vi "Substitute the assigned name for Test UI.vi"(8 "error in":errorcluster, 10 "Project Name":string, 11 "Name to VI Map":map{string, refnum<vi>}(c390)) -> (0 "error out":errorcluster)   [LabVIEW 2023, in "Plugin Generator.lvlib"]
uses:
  Plugin Generator.lvlib
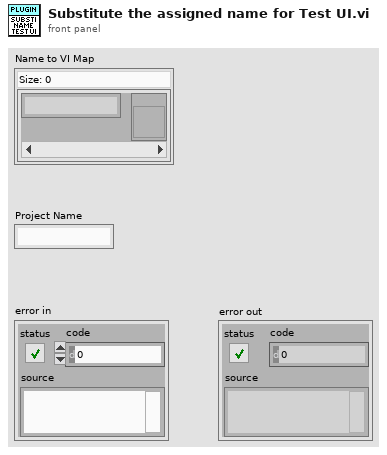
[diagram p1: front panel]
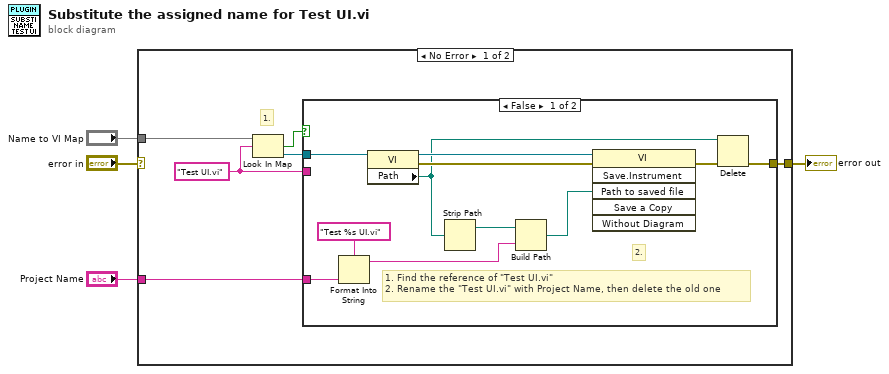
[diagram p0: block diagram]
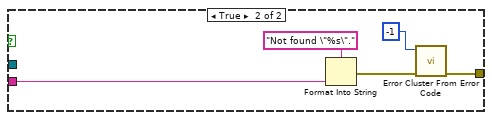
[diagram p2: hidden frame]
diagram:
  n1 = case shown="No Error" "error in" {
    selector: "error in" -> [_ w27]
    tunnel: "Project Name" -> [w10 _]
    tunnel: [w9 w27] -> w3
    tunnel: "Name to VI Map" -> [w8 _]
    frame No Error {
      w5 = "Test UI.vi" ("String")
      # "1."
      n2 = Look In Map(map=w8, key=w5) -> (key not found?=w6:bool, value=w7:refnum<vi>)  [unwired: 1 in]
      n3 = case shown="False" w6 {
        tunnel: w10 -> [w20 _]
        tunnel: [w13 w25] -> w9
        tunnel: w7 -> [w11 _]
        tunnel: w5 -> [_ w22]
        frame False {
          # "2."
          # "1. Find the reference of \"Test UI.vi\"\n2. Rename the \"Test UI.vi\" with Project Name, then delete the old one"
          n4 = Format Into String(format string="Test %s UI.vi", w20) -> (resulting string=w19:string)  [unwired: 2 in, 1 out]
          n5 = property class="VI"(reference=w11) -> (reference out=w21:refnum<vi>, error out=w15:errorcluster, "Path"=w12:path)  [unwired: 1 in]
          n6 = Strip Path(path=w12) -> (stripped path=w16:path)  [unwired: 1 out]
          n7 = Build Path(base path=w16, name or relative path=w19) -> (appended path=w17:path)
          n8 = invoke class="VI" method="Save.Instrument"(reference=w21, error in=w15, "Path to saved file"=w17) -> (error out=w14:errorcluster)  [unwired: 3 in, 5 out]
          n9 = Delete(path (use dialog)=w12, error in=w14) -> (error out=w13:errorcluster)  [unwired: 3 in, 2 out]
        }
        frame True {
          n10 = Format Into String(format string="Not found \"%s\"." ("error message (\"\")"), w22) -> (error out=w23:errorcluster)  [unwired: 2 in, 1 out]
          n11 = call <vilib>:"Error Cluster From Error Code.vi"("error in (no error)"=w23, "error code (0)"=-1) -> ("error out"=w25:errorcluster)  [unwired: 7 in]
        }
      }
    }
    frame Error {
    }
  }
  "error out" <- w3
